vi "JET_CAT_SUB.vi"() -> ()   [LabVIEW 2017]
uses:
  <vilib>/Instr/_visa.llb/VISA Configure Serial Port (Instr).vi
panel:
  in  "Send Custom Command":bool
  in  "STOP":bool
  in  "Baud Rate":u32=9600
  in  "Jetcat Port":refnum<visa-resource-name>="COM2"
  in  "shtdwn/strt":bool
  out "read buffer":string
  in  "Serial Control Toggle":bool
  in  "RPM":dbl(slide) min=0.0 max=117000.0 scale=0.0..117000.0 scale format="%#.2f"
  in  "Serial Command":string
  out "Turbine RPM":dbl
  out "Turbine Temp":dbl format="%.1f"
  out "Pump Voltage":dbl format="%.1f"
  out "Throttle Position":dbl format="%.1f"
  out "Turbine State":string
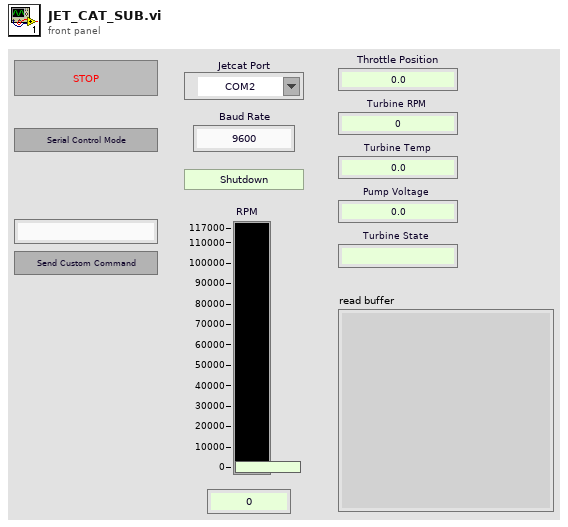
[diagram p1: front panel]
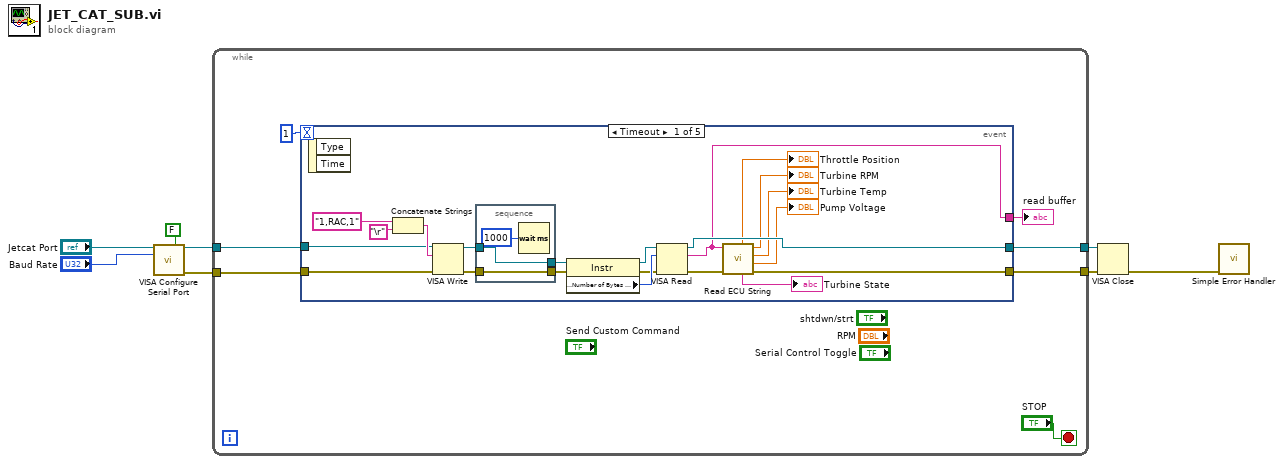
[diagram p0: block diagram]
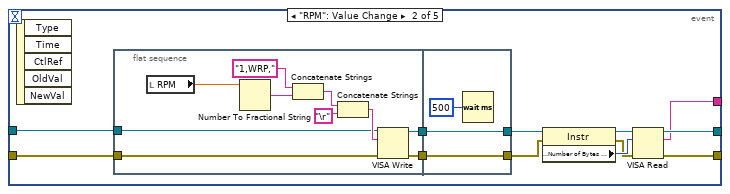
[diagram p2: hidden frame]
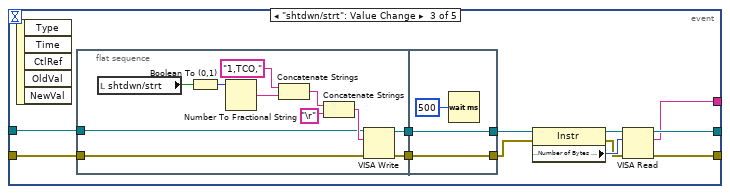
[diagram p3: hidden frame]
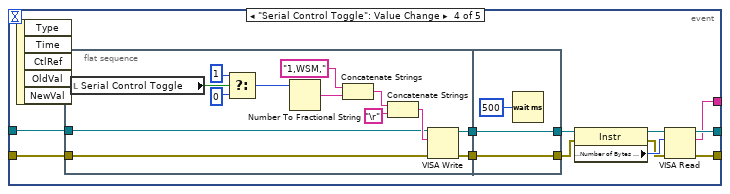
[diagram p4: hidden frame]
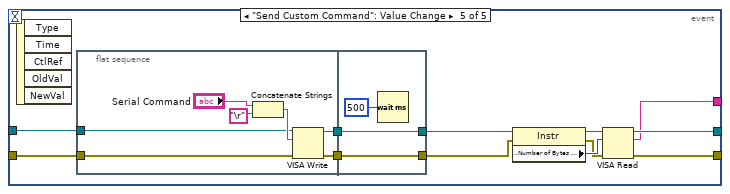
[diagram p5: hidden frame]
diagram:
  n1 = call-poly "VISA Configure Serial Port"("VISA resource name"="Jetcat Port", "Enable Termination\nChar (T)"=FALSE ("Enable Termination Char (T)"), "baud rate (9600)"="Baud Rate") -> ("VISA resource name out"=w5:refnum<visa-resource-name>, "error out"=w4:errorcluster)  [unwired: 5 in, 6 out]
  n2 = while {
    tunnel: w5 -> [w13]
    tunnel: w4 -> [w12]
    tunnel: [w11] -> w3
    tunnel: [w10] -> w2
    stop <- "STOP" stop-if-true
    n3 = event shown="[0] Timeout" {
      selector: _ -> [_ _ _ _ _]
      dyn-events: _ -> [_ _ _ _ _]
      timeout: 1 -> [_ _ _ _ _]
      tunnel: w13 -> [w24 w51 w74 w100 w128]
      tunnel: w12 -> [w25 w50 w73 w99 w127]
      tunnel: [w23 w42 w67 w93 w121] -> w11
      tunnel: [w22 w41 w66 w92 w120] -> w10
      tunnel: [w16 w40 w65 w91 w119] -> w14
      event Timeout {
        n4 = event-data() -> ()  [unwired: 1 in, 2 out]
        n5 = Concatenate Strings("1,RAC,1" ("WRITE STRING"), "\r") -> (w32:string)
        n6 = VISA Write(VISA resource name=w24, write buffer=w32, error in (no error)=w25) -> (VISA resource name out=w28:refnum<visa-resource-name>, error out=w26:errorcluster)  [unwired: 1 out]
        n7 = stacked-sequence {
          tunnel: w26 -> [w39]
          tunnel: [w39] -> w27
          tunnel: w28 -> [w38]
          tunnel: [w38] -> w29
          frame #0 {
            n8 = Wait (ms)(milliseconds to wait=u32 1000 ("delay before read (ms)")) -> ()  [unwired: 1 out]
          }
        }
        n9 = property class="Instr"(reference=w29, error in=w27) -> (reference out=w33:refnum<visa-resource-name>, error out=w34:errorcluster, "Serial Settings:Number of Bytes at Serial Port"=w35:u32)
        n10 = VISA Read(VISA resource name=w33, byte count=w35, error in (no error)=w34) -> (VISA resource name out=w23:refnum<visa-resource-name>, read buffer=w16:string, error out=w36:errorcluster)  [unwired: 1 out]
        n11 = call "Read ECU String.vi"("error in (no error)"=w36, "String"=w16) -> ("error out"=w22:errorcluster, "Pump Voltage"=→"Pump Voltage":dbl, "Turbine Temp"=→"Turbine Temp":dbl, "Turbine RPM"=→"Turbine RPM":dbl, "Turbine State"=→"Turbine State":string, "Throttle Position"=→"Throttle Position":dbl)  [unwired: 4 out]
      }
      event "RPM": Value Change {
        n12 = event-data() -> ()  [unwired: 1 in, 5 out]
        n13 = flat-sequence {
          tunnel: w51 -> [w59]
          tunnel: w50 -> [w58]
          tunnel: [w57] -> w49
          tunnel: [w56] -> w48
          tunnel: [w63] -> w43
          tunnel: [w64] -> w44
          tunnel: w49 -> [w64]
          tunnel: w48 -> [w63]
          frame #0 {
            n14 = local read "RPM"() -> (w52:dbl)
            n15 = Number To Fractional String(number=w52) -> (F-format string=w54:string)  [unwired: 3 in]
            n16 = Concatenate Strings("1,WRP," ("WRITE STRING"), w54) -> (w53:string)
            n17 = Concatenate Strings(w53, "\r") -> (w61:string)
            n18 = VISA Write(VISA resource name=w59, write buffer=w61, error in (no error)=w58) -> (VISA resource name out=w57:refnum<visa-resource-name>, error out=w56:errorcluster)  [unwired: 1 out]
          }
          frame #1 {
            n19 = Wait (ms)(milliseconds to wait=u32 500) -> ()  [unwired: 1 out]
          }
        }
        n20 = property class="Instr"(reference=w44, error in=w43) -> (reference out=w45:refnum<visa-resource-name>, error out=w46:errorcluster, "Serial Settings:Number of Bytes at Serial Port"=w47:u32)
        n21 = VISA Read(VISA resource name=w45, byte count=w47, error in (no error)=w46) -> (VISA resource name out=w42:refnum<visa-resource-name>, read buffer=w40:string, error out=w41:errorcluster)  [unwired: 1 out]
      }
      event "shtdwn/strt": Value Change {
        n22 = event-data() -> ()  [unwired: 1 in, 5 out]
        n23 = flat-sequence {
          tunnel: w74 -> [w85]
          tunnel: w73 -> [w84]
          tunnel: [w83] -> w76
          tunnel: [w82] -> w75
          tunnel: [w89] -> w68
          tunnel: [w90] -> w69
          tunnel: w76 -> [w90]
          tunnel: w75 -> [w89]
          frame #0 {
            n24 = local read "shtdwn/strt"() -> (w77:bool)
            n25 = Boolean To (0,1)(Boolean=w77) -> (0, 1=w78:i16)
            n26 = Number To Fractional String(number=w78) -> (F-format string=w80:string)  [unwired: 3 in]
            n27 = Concatenate Strings("1,TCO," ("WRITE STRING"), w80) -> (w79:string)
            n28 = Concatenate Strings(w79, "\r") -> (w87:string)
            n29 = VISA Write(VISA resource name=w85, write buffer=w87, error in (no error)=w84) -> (VISA resource name out=w83:refnum<visa-resource-name>, error out=w82:errorcluster)  [unwired: 1 out]
          }
          frame #1 {
            n30 = Wait (ms)(milliseconds to wait=u32 500) -> ()  [unwired: 1 out]
          }
        }
        n31 = property class="Instr"(reference=w69, error in=w68) -> (reference out=w70:refnum<visa-resource-name>, error out=w71:errorcluster, "Serial Settings:Number of Bytes at Serial Port"=w72:u32)
        n32 = VISA Read(VISA resource name=w70, byte count=w72, error in (no error)=w71) -> (VISA resource name out=w67:refnum<visa-resource-name>, read buffer=w65:string, error out=w66:errorcluster)  [unwired: 1 out]
      }
      event "Serial Control Toggle": Value Change {
        n33 = event-data() -> ()  [unwired: 1 in, 5 out]
        n34 = flat-sequence {
          tunnel: w100 -> [w113]
          tunnel: w99 -> [w112]
          tunnel: [w111] -> w102
          tunnel: [w110] -> w101
          tunnel: [w117] -> w94
          tunnel: [w118] -> w95
          tunnel: w102 -> [w118]
          tunnel: w101 -> [w117]
          frame #0 {
            n35 = local read "Serial Control Toggle"() -> (w103:bool)
            n36 = Select(t=1, s=w103, f=0) -> (s? t:f=w104:i32)
            n37 = Number To Fractional String(number=w104) -> (F-format string=w108:string)  [unwired: 3 in]
            n38 = Concatenate Strings("1,WSM," ("WRITE STRING"), w108) -> (w107:string)
            n39 = Concatenate Strings(w107, "\r") -> (w115:string)
            n40 = VISA Write(VISA resource name=w113, write buffer=w115, error in (no error)=w112) -> (VISA resource name out=w111:refnum<visa-resource-name>, error out=w110:errorcluster)  [unwired: 1 out]
          }
          frame #1 {
            n41 = Wait (ms)(milliseconds to wait=u32 500) -> ()  [unwired: 1 out]
          }
        }
        n42 = property class="Instr"(reference=w95, error in=w94) -> (reference out=w96:refnum<visa-resource-name>, error out=w97:errorcluster, "Serial Settings:Number of Bytes at Serial Port"=w98:u32)
        n43 = VISA Read(VISA resource name=w96, byte count=w98, error in (no error)=w97) -> (VISA resource name out=w93:refnum<visa-resource-name>, read buffer=w91:string, error out=w92:errorcluster)  [unwired: 1 out]
      }
      event "Send Custom Command": Value Change {
        n44 = event-data() -> ()  [unwired: 1 in, 5 out]
        n45 = flat-sequence {
          tunnel: w128 -> [w135]
          tunnel: w127 -> [w134]
          tunnel: [w133] -> w130
          tunnel: [w132] -> w129
          tunnel: w130 -> [w139]
          tunnel: w129 -> [w138]
          tunnel: [w139] -> w123
          tunnel: [w138] -> w122
          frame #0 {
            n46 = Concatenate Strings("Serial Command", "\r") -> (w137:string)
            n47 = VISA Write(VISA resource name=w135, write buffer=w137, error in (no error)=w134) -> (VISA resource name out=w133:refnum<visa-resource-name>, error out=w132:errorcluster)  [unwired: 1 out]
          }
          frame #1 {
            n48 = Wait (ms)(milliseconds to wait=u32 500) -> ()  [unwired: 1 out]
          }
        }
        n49 = property class="Instr"(reference=w123, error in=w122) -> (reference out=w124:refnum<visa-resource-name>, error out=w125:errorcluster, "Serial Settings:Number of Bytes at Serial Port"=w126:u32)
        n50 = VISA Read(VISA resource name=w124, byte count=w126, error in (no error)=w125) -> (VISA resource name out=w121:refnum<visa-resource-name>, read buffer=w119:string, error out=w120:errorcluster)  [unwired: 1 out]
      }
    }
    "read buffer" <- w14
  }
  n51 = VISA Close(VISA resource name=w3, error in (no error)=w2) -> (error out=w1:errorcluster)
  n52 = call <vilib>:"Simple Error Handler.vi"("error in (no error)"=w1) -> ()  [unwired: 4 in, 5 out]
